vi "FLIN Read Data.vi"(9 "pData":u8[](array[numeric])=array[4097 elements], 10 "LINIndex":u8, 11 "DevHandle":i32) -> (1 "pData out":u8[](array[numeric]), 3 "function return":i32)   [LabVIEW 2010, in "usb2fast_lin.lvlib"]
doc: "int WINAPI FLIN_ReadData(int DevHandle,unsigned char LINIndex,unsigned char *pData);"
uses:
  usb2fast_lin.lvlib
  USB2XXX/trunk/USB2XXX/USB2XXX/vs2010/Release/USB2XXX.dll
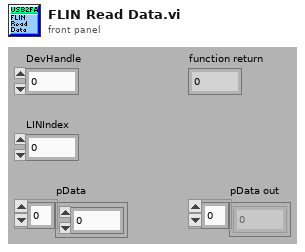
[diagram p1: front panel]
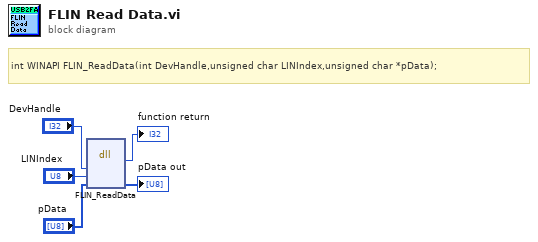
[diagram p0: block diagram]
diagram:
  # "int WINAPI FLIN_ReadData(int DevHandle,unsigned char LINIndex,unsigned char *pData);"
  n1 = dll-call lib="E:/Projects/USB2XXX/trunk/USB2XXX/USB2XXX/vs2010/Release/USB2XXX.*" fn="FLIN_ReadData"("DevHandle"="DevHandle", "LINIndex"="LINIndex", "pData"="pData") -> (→"function return":i32, "pData"=→"pData out":u8[])  [unwired: 5 in, 2 out]
